vi "Autonomous Independent.vi"() -> ()   [LabVIEW 2016]
doc: "This VI is called when autonomous begins, and will automatically be terminated when autonomous ends. You can carry out timed or sensor driven robot movement independently without needing to return to the caller."
uses:
  <vilib>/Rock Robotics/Network Tables/NT Read Number.vi
  Global 2.vi
  Systems/Global 1.vi
panel:
  out "Numeric":i32=5
  out "Gyro":dbl=-2.5767482712972
  in  "Oscillate effort":dbl=0.25 format="%#_13g"
  out "Auto Mode":dbl
  in  "Auton_Modes":T1(array[cluster])=[{"Actions"=[{"Effort"=0.55, "Duration"=3.5, "Action"=enum."Vision Correction", "Encoder"=0.0, "Condition"=FALSE}, {"Effort"=0.0, "Duration"=0.0, "Action"=enum."Nothing", "Encoder"=0.0, "Condition"=FALSE}]}, {"Actions"=[{"Effort"=0.53, "Duration"=1.0, "Action"=enum."Shoot", "Encoder"=6.462, "Condition"=TRUE}, {"Effort"=0.0, "Duration"=3.0, "Action"=enum."Index", "Encoder"=0.0, "Condition"=FALSE}, {"Effort"=0.3, "Duration"=2.0, "Action"=enum."Turn", "Encoder"=38.0, "Condition"=FALSE}, {"Effort"=0.3, "Duration"=5.0, "Action"=enum."Drive", "Encoder"=0.0, "Condition"=TRUE}, {"Effort"=0.25, "Duration"=0.0, "Action"=enum."Nothing", "Encoder"=57.0, "Condition"=FALSE}, {"Effort"=-0.25, "Duration"=0.0, "Action"=enum."Nothing", "Encoder"=0.0, "Condition"=FALSE}, {"Effort"=1.0, "Duration"=0.0, "Action"=enum."Nothing", "Encoder"=0.0, "Condition"=FALSE}, {"Effort"=0.25, "Duration"=0.0, "Action"=enum."Nothing", "Encoder"=0.0, "Condition"=FALSE}]}, {"Actions"=[{"Effort"=0.0, "Duration"=0.1, "Action"=enum."Drive Encoder Reset", "Encoder"=0.0, "Condition"=FALSE}, {"Effort"=0.0, "Duration"=0.1, "Action"=enum."Gyro Reset", "Encoder"=0.0, "Condition"=FALSE}, {"Effort"=0.3, "Duration"=4.0, "Action"=enum."Drive", "Encoder"=60.0, "Condition"=FALSE}, {"Effort"=1.0, "Duration"=1.0, "Action"=enum."Gear0", "Encoder"=0.0, "Condition"=FALSE}, {"Effort"=1.0, "Duration"=0.0, "Action"=enum."Nothing", "Encoder"=0.0, "Condition"=FALSE}, {"Effort"=1.0, "Duration"=0.0, "Action"=enum."Nothing", "Encoder"=0.0, "Condition"=FALSE}, {"Effort"=0.0, "Duration"=0.0, "Action"=enum."Drive Encoder Reset", "Encoder"=0.0, "Condition"=FALSE}, {"Effort"=0.0, "Duration"=0.0, "Action"=enum."Nothing", "Encoder"=0.0, "Condition"=FALSE}, {"Effort"=0.0, "Duration"=0.0, "Action"=enum."Nothing", "Encoder"=0.0, "Condition"=FALSE}, {"Effort"=-0.2, "Duration"=10000.0, "Action"=enum."Drive", "Encoder"=24.0, "Condition"=FALSE}, {"Effort"=0.0, "Duration"=0.0, "Action"=enum."Drive Encoder Reset", "Encoder"=0.0, "Condition"=FALSE}, {"Effort"=-0.25, "Duration"=0.0, "Action"=enum."Nothing", "Encoder"=12.0, "Condition"=FALSE}]}, {"Actions"=[{"Effort"=0.0, "Duration"=0.1, "Action"=enum."Drive Encoder Reset", "Encoder"=6.462, "Condition"=FALSE}, {"Effort"=0.0, "Duration"=0.1, "Action"=enum."Gyro Reset", "Encoder"=0.0, "Condition"=FALSE}, {"Effort"=-0.25, "Duration"=1.0, "Action"=enum."Drive", "Encoder"=6.462, "Condition"=FALSE}, {"Effort"=0.0, "Duration"=0.1, "Action"=enum."Gyro Reset", "Encoder"=0.0, "Condition"=FALSE}, {"Effort"=-0.25, "Duration"=0.0, "Action"=enum."Turn", "Encoder"=0.0, "Condition"=FALSE}, {"Effort"=-0.25, "Duration"=0.0, "Action"=enum."Drive", "Encoder"=7.5, "Condition"=FALSE}, {"Effort"=-1.0, "Duration"=0.0, "Action"=enum."Gear0", "Encoder"=0.0, "Condition"=FALSE}, {"Effort"=0.25, "Duration"=0.0, "Action"=enum."Drive", "Encoder"=3.0, "Condition"=FALSE}]}, {"Actions"=[{"Effort"=0.0, "Duration"=0.1, "Action"=enum."Drive Encoder Reset", "Encoder"=6.462, "Condition"=FALSE}, {"Effort"=0.0, "Duration"=0.1, "Action"=enum."Gyro Reset", "Encoder"=0.0, "Condition"=FALSE}, {"Effort"=-0.25, "Duration"=1.0, "Action"=enum."Drive", "Encoder"=6.462, "Condition"=FALSE}, {"Effort"=0.0, "Duration"=0.1, "Action"=enum."Gyro Reset", "Encoder"=0.0, "Condition"=FALSE}, {"Effort"=-0.25, "Duration"=0.0, "Action"=enum."Turn", "Encoder"=0.0, "Condition"=FALSE}, {"Effort"=-0.25, "Duration"=0.0, "Action"=enum."Drive", "Encoder"=7.5, "Condition"=FALSE}, {"Effort"=-1.0, "Duration"=0.0, "Action"=enum."Gear0", "Encoder"=0.0, "Condition"=FALSE}, {"Effort"=0.25, "Duration"=0.0, "Action"=enum."Drive", "Encoder"=3.0, "Condition"=FALSE}]}, {"Actions"=[{"Effort"=0.0, "Duration"=0.1, "Action"=enum."Drive Encoder Reset", "Encoder"=0.0, "Condition"=FALSE}, {"Effort"=0.0, "Duration"=0.1, "Action"=enum."Gyro Reset", "Encoder"=0.0, "Condition"=FALSE}, {"Effort"=0.25, "Duration"=1.0, "Action"=enum."Drive", "Encoder"=6.462, "Condition"=FALSE}, {"Effort"=1.0, "Duration"=0.1, "Action"=enum."Gyro Reset", "Encoder"=0.0, "Condition"=FALSE}, {"Effort"=0.25, "Duration"=0.0, "Action"=enum."Turn", "Encoder"=0.0, "Condition"=FALSE}, {"Effort"=0.25, "Duration"=0.0, "Action"=enum."Drive", "Encoder"=7.5, "Condition"=FALSE}, {"Effort"=1.0, "Duration"=0.0, "Action"=enum."Gear0", "Encoder"=0.0, "Condition"=FALSE}, {"Effort"=-0.25, "Duration"=0.0, "Action"=enum."Drive", "Encoder"=3.0, "Condition"=FALSE}]}, {"Actions"=[{"Effort"=0.0, "Duration"=0.1, "Action"=enum."Nothing", "Encoder"=0.0, "Condition"=FALSE}, {"Effort"=0.0, "Duration"=0.1, "Action"=enum."Gyro Reset", "Encoder"=0.0, "Condition"=FALSE}, {"Effort"=0.25, "Duration"=5.0, "Action"=enum."Drive", "Encoder"=60000.0, "Condition"=TRUE}, {"Effort"=0.75, "Duration"=1.0, "Action"=enum."Nothing", "Encoder"=0.0, "Condition"=FALSE}, {"Effort"=0.0, "Duration"=1.0, "Action"=enum."Nothing", "Encoder"=0.0, "Condition"=FALSE}, {"Effort"=0.0, "Duration"=0.0, "Action"=enum."Nothing", "Encoder"=0.0, "Condition"=FALSE}]}, {"Actions"=[{"Effort"=0.0, "Duration"=0.1, "Action"=enum."Drive Encoder Reset", "Encoder"=0.0, "Condition"=FALSE}, {"Effort"=0.0, "Duration"=0.1, "Action"=enum."Gyro Reset", "Encoder"=0.0, "Condition"=FALSE}, {"Effort"=0.3, "Duration"=0.0, "Action"=enum."Drive", "Encoder"=24.0, "Condition"=FALSE}, {"Effort"=0.3, "Duration"=3.0, "Action"=enum."Nothing", "Encoder"=0.0, "Condition"=FALSE}, {"Effort"=0.3, "Duration"=2.0, "Action"=enum."Vision Correction", "Encoder"=30.0, "Condition"=FALSE}, {"Effort"=0.2, "Duration"=1.0, "Action"=enum."Drive", "Encoder"=18.5, "Condition"=TRUE}, {"Effort"=1.0, "Duration"=0.0, "Action"=enum."Gear0", "Encoder"=0.0, "Condition"=FALSE}, {"Effort"=-0.2, "Duration"=1.3, "Action"=enum."Drive", "Encoder"=30.0, "Condition"=TRUE}, {"Effort"=0.0, "Duration"=3.0, "Action"=enum."Nothing", "Encoder"=0.0, "Condition"=FALSE}, {"Effort"=0.03, "Duration"=0.0, "Action"=enum."Turn", "Encoder"=0.0, "Condition"=FALSE}, {"Effort"=0.0, "Duration"=0.0, "Action"=enum."Drive", "Encoder"=0.0, "Condition"=FALSE}]}, {"Actions"=[{"Effort"=0.0, "Duration"=0.0, "Action"=enum."Nothing", "Encoder"=0.0, "Condition"=FALSE}]}, {"Actions"=[{"Effort"=0.0, "Duration"=2.5, "Action"=enum."Shoot", "Encoder"=0.0, "Condition"=FALSE}, {"Effort"=0.0, "Duration"=5.0, "Action"=enum."Index", "Encoder"=0.0, "Condition"=FALSE}, {"Effort"=0.25, "Duration"=3.5, "Action"=enum."Nothing", "Encoder"=88.0, "Condition"=FALSE}, {"Effort"=1.0, "Duration"=1.0, "Action"=enum."Nothing", "Encoder"=0.0, "Condition"=FALSE}, {"Effort"=1.0, "Duration"=1.0, "Action"=enum."Nothing", "Encoder"=0.0, "Condition"=FALSE}, {"Effort"=1.0, "Duration"=0.5, "Action"=enum."Nothing", "Encoder"=0.0, "Condition"=FALSE}, {"Effort"=0.0, "Duration"=0.0, "Action"=enum."Nothing", "Encoder"=0.0, "Condition"=FALSE}, {"Effort"=-0.25, "Duration"=0.0, "Action"=enum."Nothing", "Encoder"=3.0, "Condition"=FALSE}, {"Effort"=0.0, "Duration"=0.0, "Action"=enum."Nothing", "Encoder"=0.0, "Condition"=FALSE}, {"Effort"=0.25, "Duration"=0.0, "Action"=enum."Nothing", "Encoder"=24.0, "Condition"=FALSE}, {"Effort"=0.0, "Duration"=0.0, "Action"=enum."Nothing", "Encoder"=0.0, "Condition"=FALSE}, {"Effort"=-0.25, "Duration"=0.0, "Action"=enum."Nothing", "Encoder"=12.0, "Condition"=FALSE}]}, {"Actions"=[{"Effort"=0.0, "Duration"=0.1, "Action"=enum."Drive Encoder Reset", "Encoder"=0.0, "Condition"=FALSE}, {"Effort"=0.0, "Duration"=1.0, "Action"=enum."Gyro Reset", "Encoder"=0.0, "Condition"=FALSE}, {"Effort"=0.3, "Duration"=1.4, "Action"=enum."Drive", "Encoder"=88.0, "Condition"=FALSE}, {"Effort"=0.3, "Duration"=3.0, "Action"=enum."Turn", "Encoder"=2.0, "Condition"=FALSE}, {"Effort"=1.0, "Duration"=1.0, "Action"=enum."Nothing", "Encoder"=0.0, "Condition"=FALSE}, {"Effort"=1.0, "Duration"=1.0, "Action"=enum."Nothing", "Encoder"=0.0, "Condition"=FALSE}, {"Effort"=0.0, "Duration"=0.0, "Action"=enum."Nothing", "Encoder"=0.0, "Condition"=FALSE}, {"Effort"=-0.25, "Duration"=0.0, "Action"=enum."Nothing", "Encoder"=3.0, "Condition"=FALSE}, {"Effort"=0.0, "Duration"=0.0, "Action"=enum."Nothing", "Encoder"=0.0, "Condition"=FALSE}, {"Effort"=0.25, "Duration"=0.0, "Action"=enum."Nothing", "Encoder"=24.0, "Condition"=FALSE}, {"Effort"=0.0, "Duration"=0.0, "Action"=enum."Nothing", "Encoder"=0.0, "Condition"=FALSE}, {"Effort"=-0.25, "Duration"=0.0, "Action"=enum."Nothing", "Encoder"=12.0, "Condition"=FALSE}]}, {"Actions"=[{"Effort"=0.0, "Duration"=1.0, "Action"=enum."Drive Encoder Reset", "Encoder"=0.0, "Condition"=FALSE}, {"Effort"=0.0, "Duration"=1.0, "Action"=enum."Shoot", "Encoder"=0.0, "Condition"=FALSE}, {"Effort"=0.25, "Duration"=5.0, "Action"=enum."Index", "Encoder"=88.0, "Condition"=FALSE}, {"Effort"=1.0, "Duration"=1.0, "Action"=enum."Nothing", "Encoder"=0.0, "Condition"=FALSE}, {"Effort"=1.0, "Duration"=1.0, "Action"=enum."Nothing", "Encoder"=0.0, "Condition"=FALSE}, {"Effort"=1.0, "Duration"=0.5, "Action"=enum."Nothing", "Encoder"=0.0, "Condition"=FALSE}, {"Effort"=0.0, "Duration"=0.0, "Action"=enum."Nothing", "Encoder"=0.0, "Condition"=FALSE}, {"Effort"=-0.25, "Duration"=0.0, "Action"=enum."Nothing", "Encoder"=3.0, "Condition"=FALSE}, {"Effort"=0.0, "Duration"=0.0, "Action"=enum."Nothing", "Encoder"=0.0, "Condition"=FALSE}, {"Effort"=0.25, "Duration"=0.0, "Action"=enum."Nothing", "Encoder"=24.0, "Condition"=FALSE}, {"Effort"=0.0, "Duration"=0.0, "Action"=enum."Nothing", "Encoder"=0.0, "Condition"=FALSE}, {"Effort"=-0.25, "Duration"=0.0, "Action"=enum."Nothing", "Encoder"=12.0, "Condition"=FALSE}]}, {"Actions"=[{"Effort"=0.0, "Duration"=0.1, "Action"=enum."Drive Encoder Reset", "Encoder"=0.0, "Condition"=FALSE}, {"Effort"=0.0, "Duration"=1.0, "Action"=enum."Gyro Reset", "Encoder"=0.0, "Condition"=FALSE}, {"Effort"=0.3, "Duration"=1.4, "Action"=enum."Drive", "Encoder"=88.0, "Condition"=FALSE}, {"Effort"=0.3, "Duration"=4.0, "Action"=enum."Turn", "Encoder"=0.0, "Condition"=FALSE}, {"Effort"=1.0, "Duration"=1.0, "Action"=enum."Nothing", "Encoder"=0.0, "Condition"=FALSE}, {"Effort"=1.0, "Duration"=0.5, "Action"=enum."Nothing", "Encoder"=0.0, "Condition"=FALSE}, {"Effort"=0.0, "Duration"=0.0, "Action"=enum."Nothing", "Encoder"=0.0, "Condition"=FALSE}, {"Effort"=0.3, "Duration"=0.5, "Action"=enum."Nothing", "Encoder"=24.0, "Condition"=TRUE}, {"Effort"=0.0, "Duration"=0.0, "Action"=enum."Nothing", "Encoder"=0.0, "Condition"=FALSE}, {"Effort"=-0.2, "Duration"=2.0, "Action"=enum."Nothing", "Encoder"=24.0, "Condition"=TRUE}, {"Effort"=0.0, "Duration"=0.0, "Action"=enum."Nothing", "Encoder"=0.0, "Condition"=FALSE}, {"Effort"=-0.25, "Duration"=0.0, "Action"=enum."Nothing", "Encoder"=12.0, "Condition"=FALSE}]}]
  # "Nothing"
  # "Boiler Right Right side gear"
  # "Middle Gear"
  # "Boiler Right Left Side Gear"
  # "Boiler Left RightSide Gear"
  # "Boiler Left Left Side Gear"
  # "Drive"
  # "Vision Correction"
  # "Hopper"
  # "10 ball"
  # "Farside"
  # "Boilerside-10 ball"
  # "Auto 5"
  # "Auto 6"
  # "Auto 6"
  # "Auto 7"
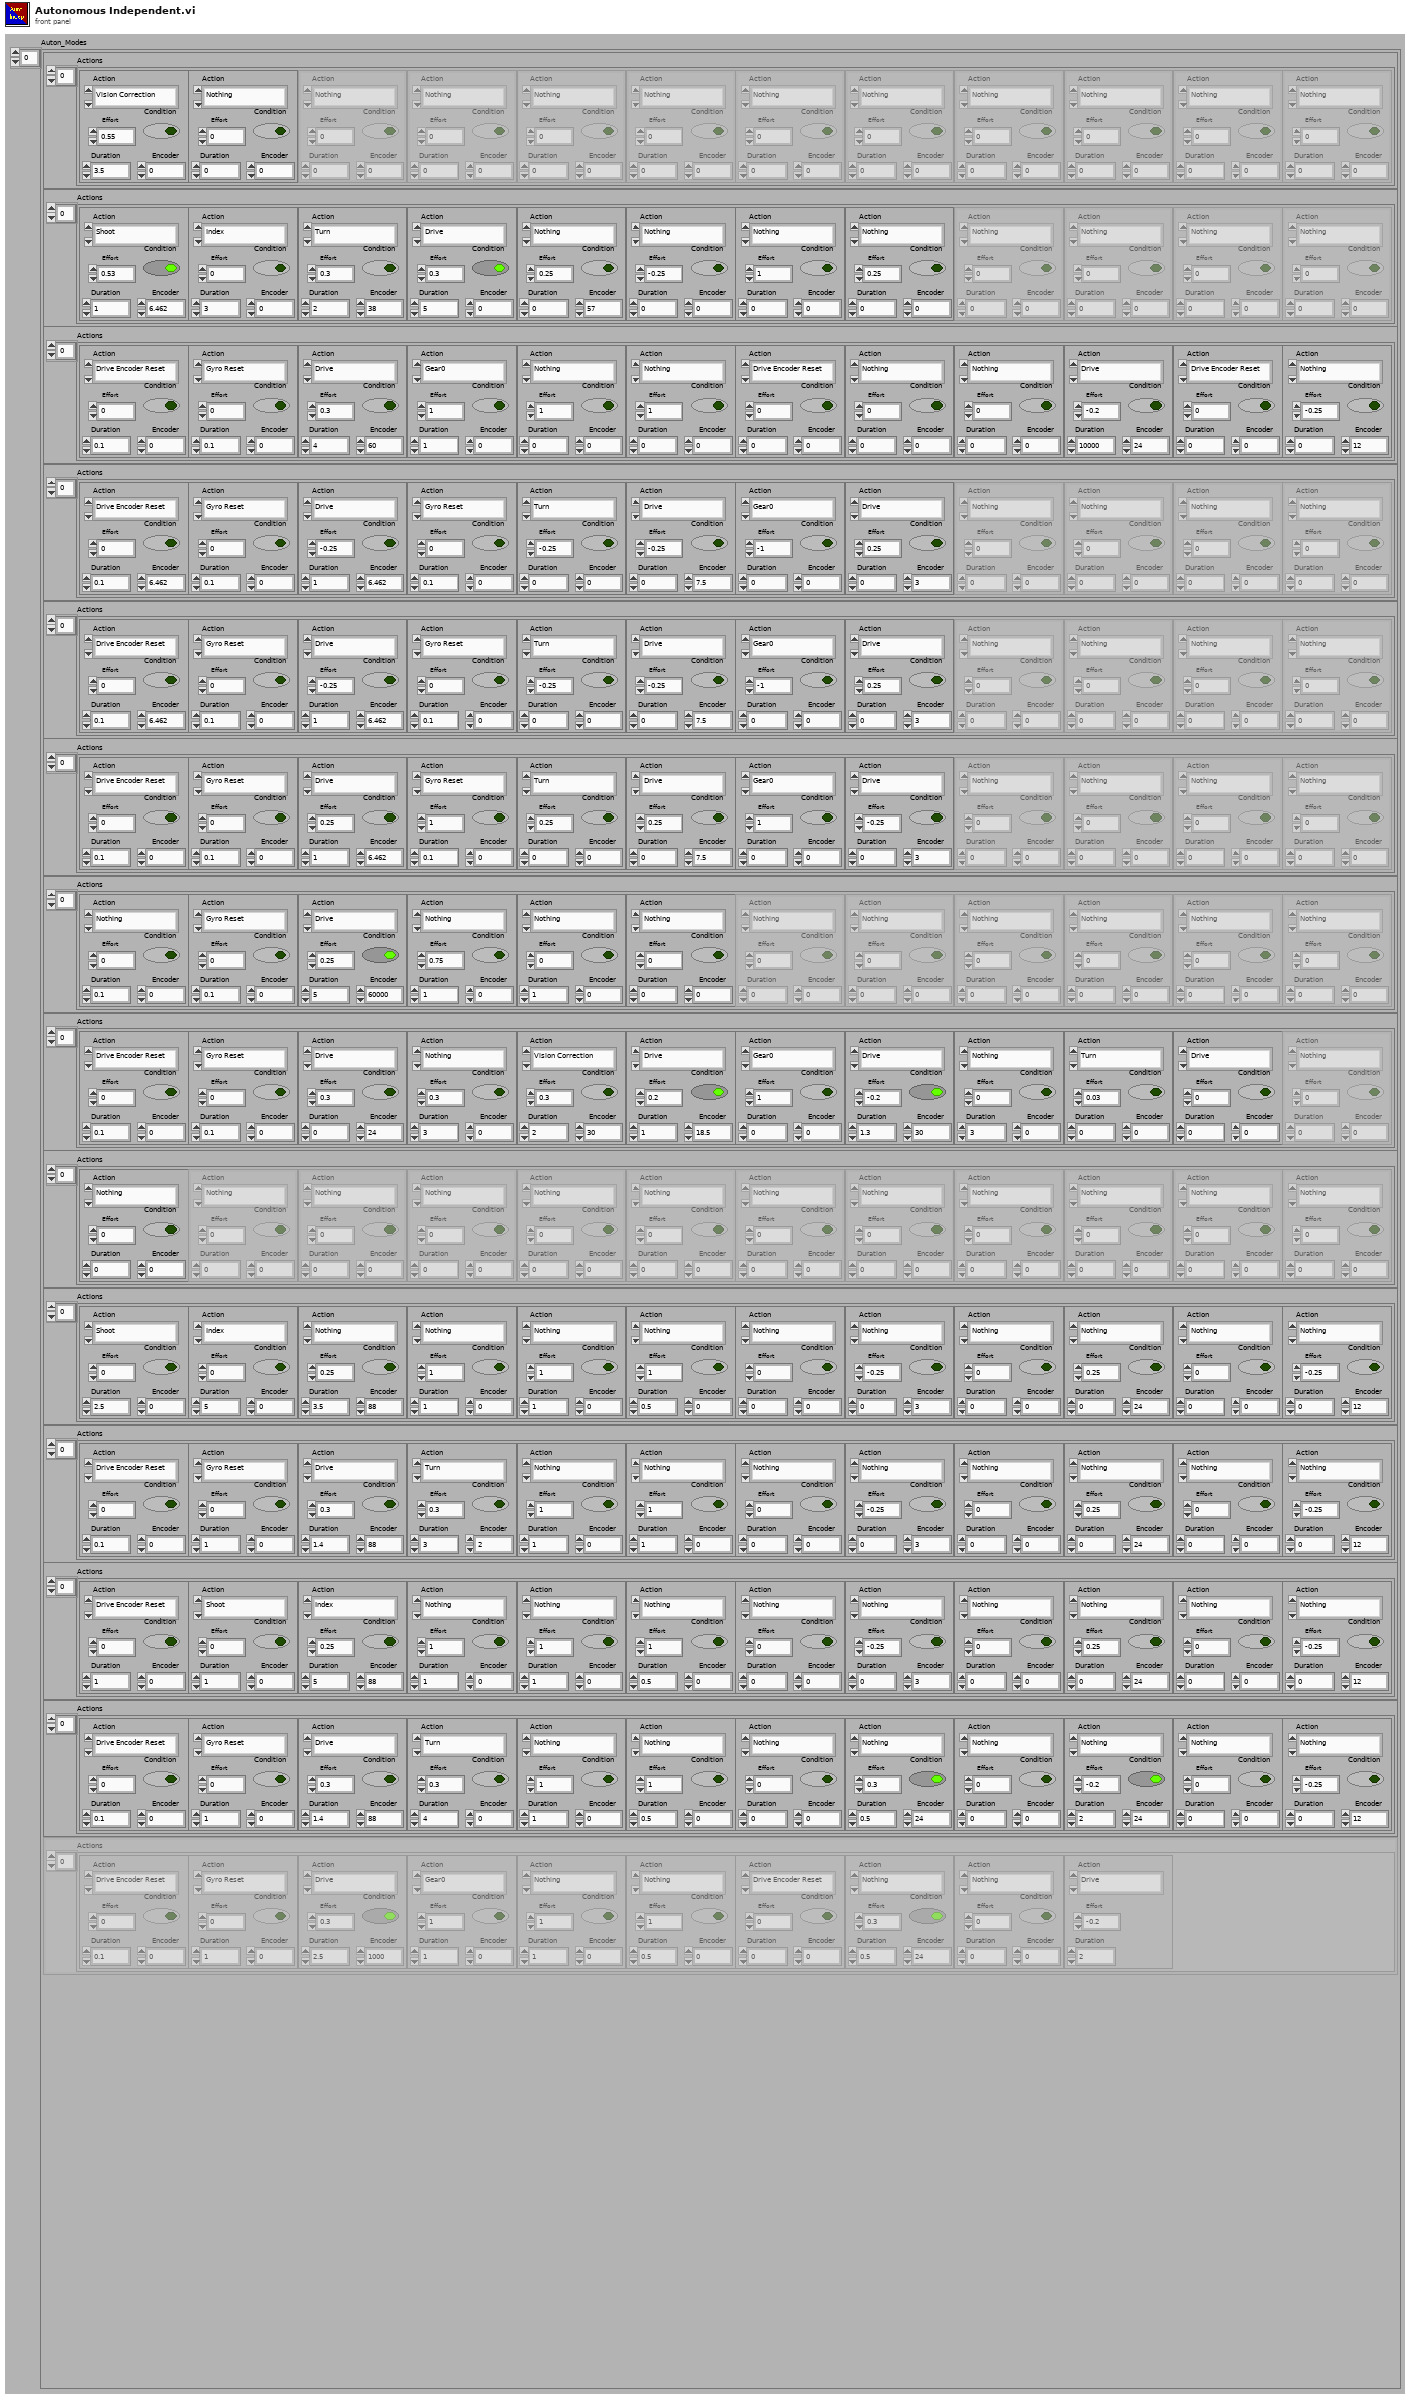
[diagram p1: front panel]
types:
  T1 = cluster{"Actions":cluster{"Effort":dbl, "Duration":dbl, "Action":enum16{"Nothing", "Drive", "Vision Correction", "Turn", "Gear0", "Gear1", "Climb", "Intake", "Index", "Shoot", "Test", "Drive Encoder Reset", "Gyro Reset"}, "Encoder":dbl, "Condition":bool}[]}[]
  T2 = cluster{"Actions":cluster{"Effort":dbl, "Duration":dbl, "Action":enum16{"Nothing", "Drive", "Vision Correction", "Turn", "Gear0", "Gear1", "Climb", "Intake", "Index", "Shoot", "Test", "Drive Encoder Reset", "Gyro Reset"}, "Encoder":dbl, "Condition":bool}[]}
  T3 = cluster{"Effort":dbl, "Duration":dbl, "Action":enum16{"Nothing", "Drive", "Vision Correction", "Turn", "Gear0", "Gear1", "Climb", "Intake", "Index", "Shoot", "Test", "Drive Encoder Reset", "Gyro Reset"}, "Encoder":dbl, "Condition":bool}[]
  T4 = enum16{"Nothing", "Drive", "Vision Correction", "Turn", "Gear0", "Gear1", "Climb", "Intake", "Index", "Shoot", "Test", "Drive Encoder Reset", "Gyro Reset"}
  T5 = typedef "WPI_MotorControlDeviceRef.ctl" = cluster{"DeviceStatus":errorcluster, "Type":T6, "PWM":cluster{"PWM Channel":T7, "DeadBand":T8}, "CAN":cluster{"Device Number":u8, "SetOutput VI Ref":variant, "GetOutput VI Ref":variant, "Enable VI Ref":variant, "Disable VI Ref":variant, "Data":variant}, "Invert":bool}
  T6 = typedef "WPI_MotorControlType.ctl" = enum16{"PWM", "CAN"}
  T7 = typedef "FPGA_DIOPWMChannel.ctl" = enum8{"PWM 0", "PWM 1", "PWM 2", "PWM 3", "PWM 4", "PWM 5", "PWM 6", "PWM 7", "PWM 8", "PWM 9", "PWM MXP 0", "PWM MXP 1", "PWM MXP 2", "PWM MXP 3", "PWM MXP 4", "PWM MXP 5", "PWM MXP 6", "PWM MXP 7", "PWM MXP 8", "PWM MXP 9", "Invalid"}
  T8 = typedef "WPI_PWMDeadband.ctl" = cluster{"Name":string, "maxPositivePwm":i32, "minPositivePwm":i32, "centerPwm":i32, "maxNegativePwm":i32, "minNegativePwm":i32, "angularRange":u16}
  T9 = typedef "WPI_CANTalonSRX_GlobalStatus.ctl" = cluster{"Applied Throttle":dbl, "Module Enabled":bool, "CAN Error":errorcluster, "Closed Loop Error":dbl, "Forward Limit Switch Closed":bool, "Reverse Limit Switch Closed":bool, "Sensor Position":dbl, "Sensor Velocity":dbl, "Current":dbl, "Sticky Fault - Over Temp":bool, "Sticky Fault - Under Voltage":bool, "Sticky Fault - Forward Limit":bool, "Sticky Fault - Reverse Limit":bool, "Sticky Fault - Forward Soft Limit":bool, "Sticky Fault - Reverse Soft Limit":bool, "Brake is Enabled":bool, "Encoder Position":dbl, "Encoder Velocity":dbl, "Encoder Index Count":dbl, "Encoder A Pin State":bool, "Encoder B Pin State":bool, "Encoder Index Pin State":bool, "Analog In":dbl, "Analog In Velocity":dbl, "Temperature (C)":dbl, "Battery Voltage":dbl, "Control 5 Is Supported":bool, "Current Profile Slot Select":dbl, "Pos Div 8":bool, "Vel Div 4":bool, "Pulse Width Position":i32, "Pulse Width Velocity":i32, "Pulse Width Rise To Rise (us)":i32, "Pulse Width Rise To Fall (us)":i32, "Mot Prof Active Is Under Run":bool, "Mot Prof Active Has Under Run":bool, "Mot Prof Active Is Last":bool, "Mot Prof Active Velocity Only":bool, "Mot Prof Active Is Valid":bool, "Mot Prof Buffer Is Full":bool, "Mot Prof Active Profile Slot Select":i32, "Mot Prof NextID":i32, "Mot Prof Count":i32, "Mot Prof Active Velocity":dbl, "Mot Prof Active Position":dbl, "Mot Prof Output Enable":i32}
  T10 = typedef "WPI_GyroDevRef.ctl" = cluster{"DevStatus":errorcluster, "Analog Channel":T11, "Offset":dbl, "Gain (VoltsPerDegree/Second)":dbl, "Gyro Type":enum16{"Analog", "XRS450"}, "Handle":i32, "SPI Bus":T12, "Device Found":bool, "Sample Rate":dbl, "Calibrate On Open":bool}
  T11 = typedef "FPGA_AIChannel.ctl" = enum8{"AI 0", "AI 1", "AI 2", "AI 3", "AI MXP 0", "AI MXP 1", "AI MXP 2", "AI MXP 3", "Invalid"}
  T12 = typedef "spi_bus.ctl" = enum16{"SPI On-Board, CS0", "SPI On-Board, CS1", "SPI On-Board, CS2", "SPI On-Board, CS3", "SPI MXP", "Invalid"}
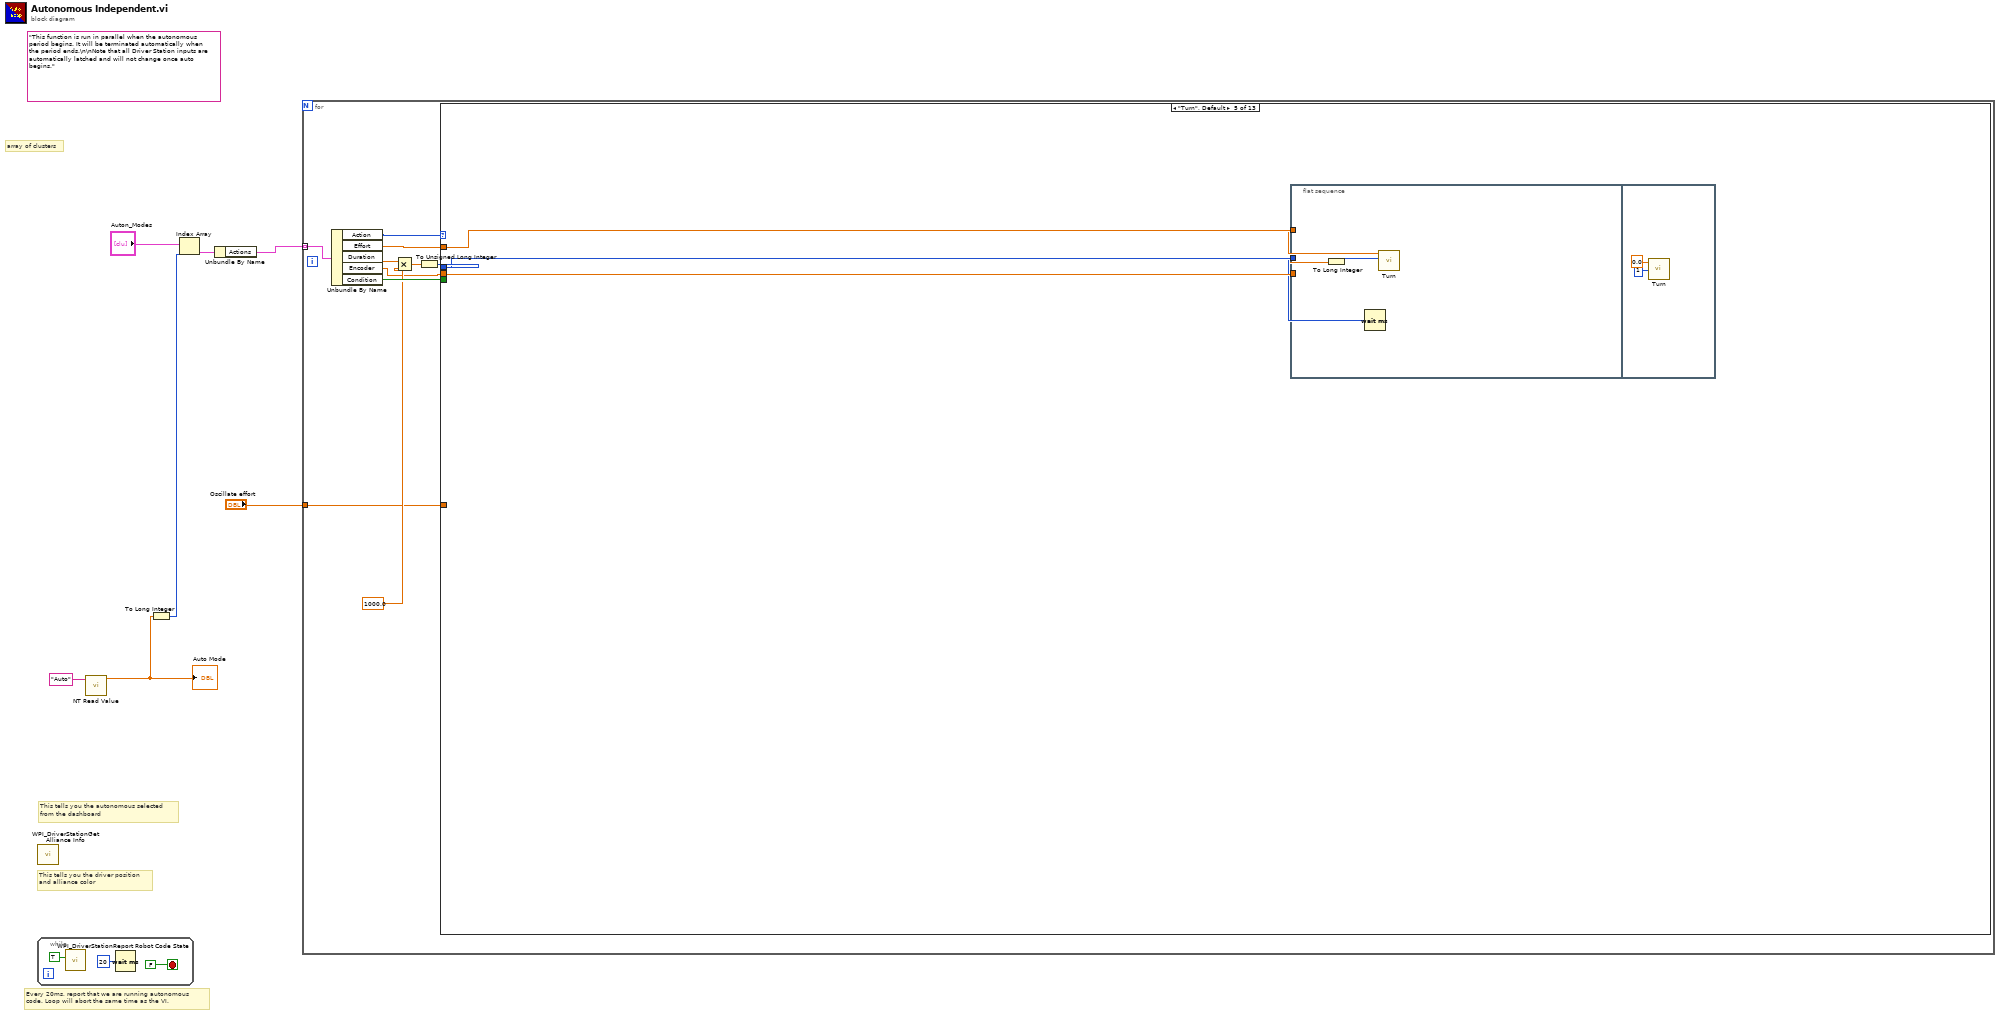
[diagram p0: block diagram]
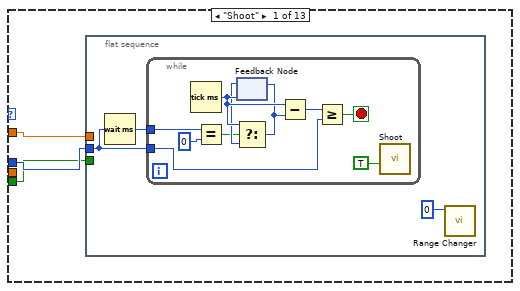
[diagram p2: hidden frame]
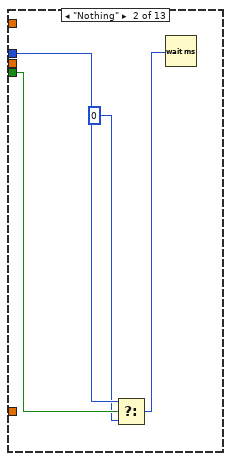
[diagram p3: hidden frame]
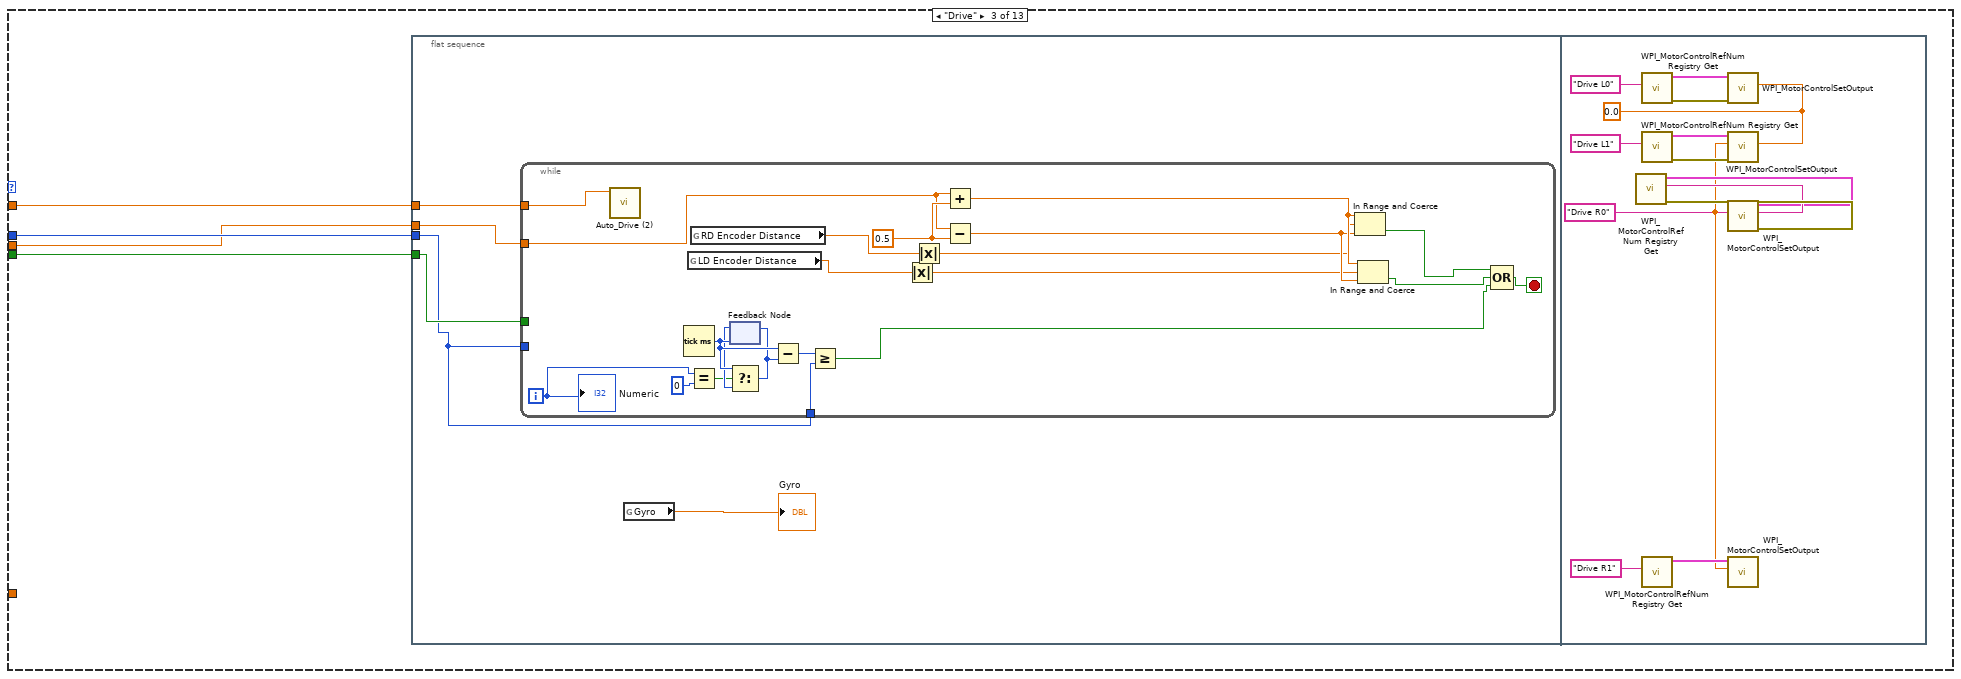
[diagram p4: hidden frame]
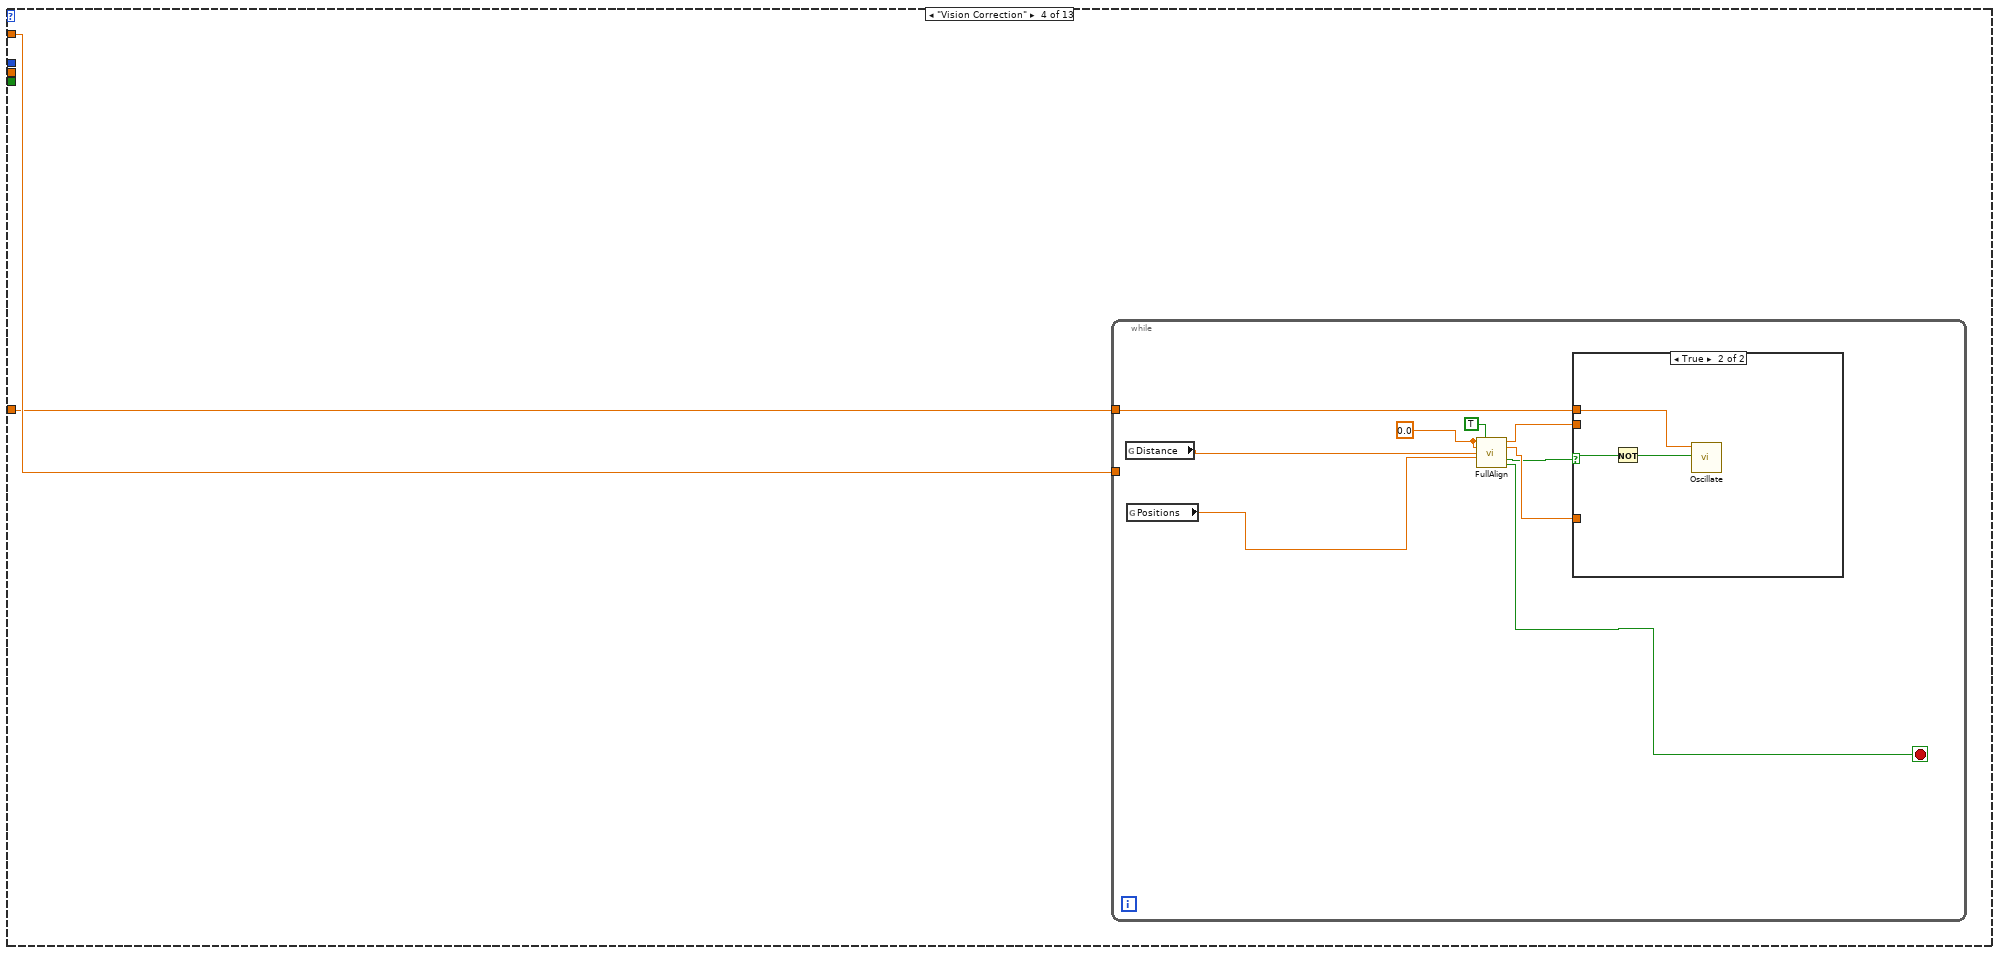
[diagram p5: hidden frame]
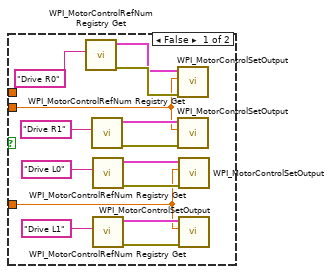
[diagram p6: hidden frame]
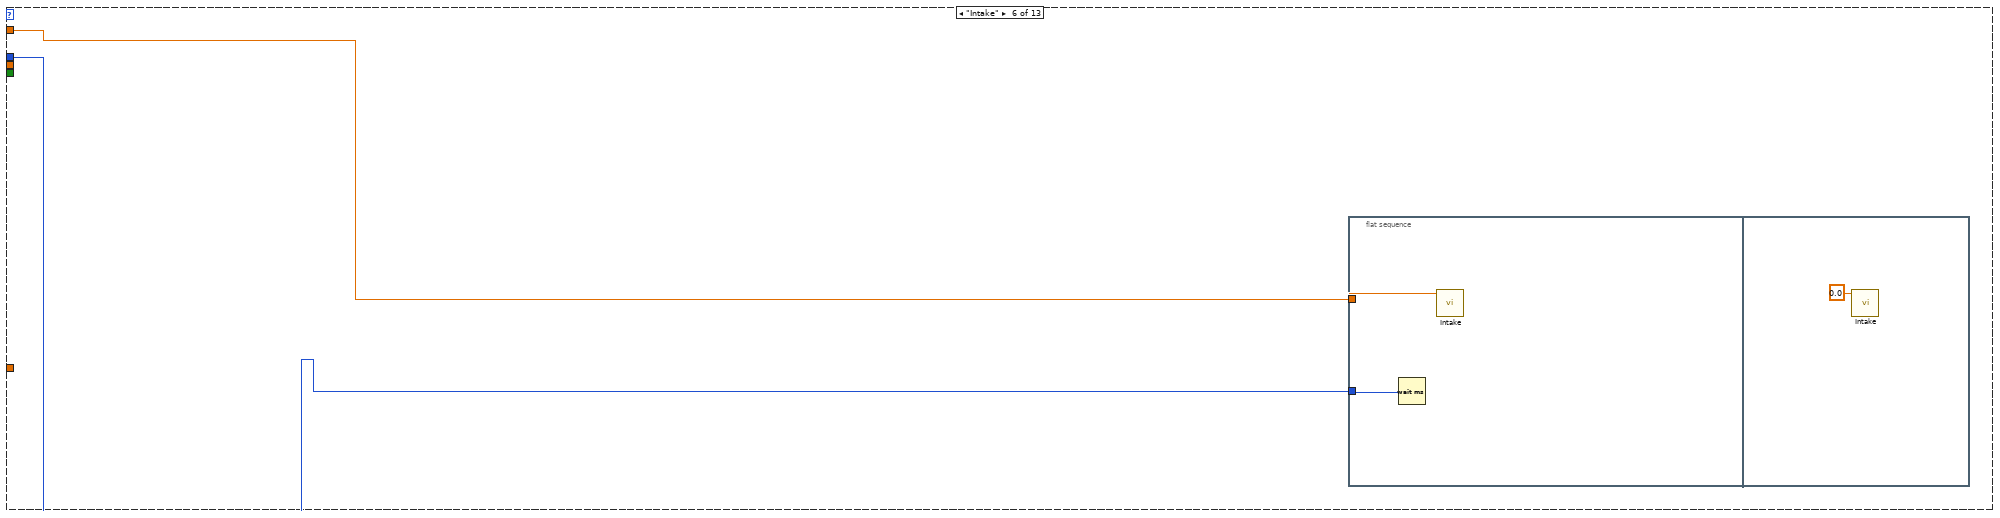
[diagram p7: hidden frame]
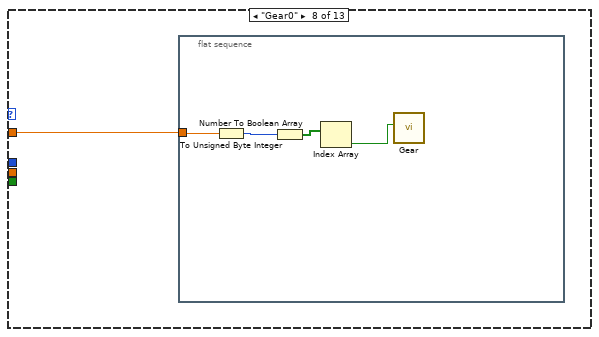
[diagram p9: hidden frame]
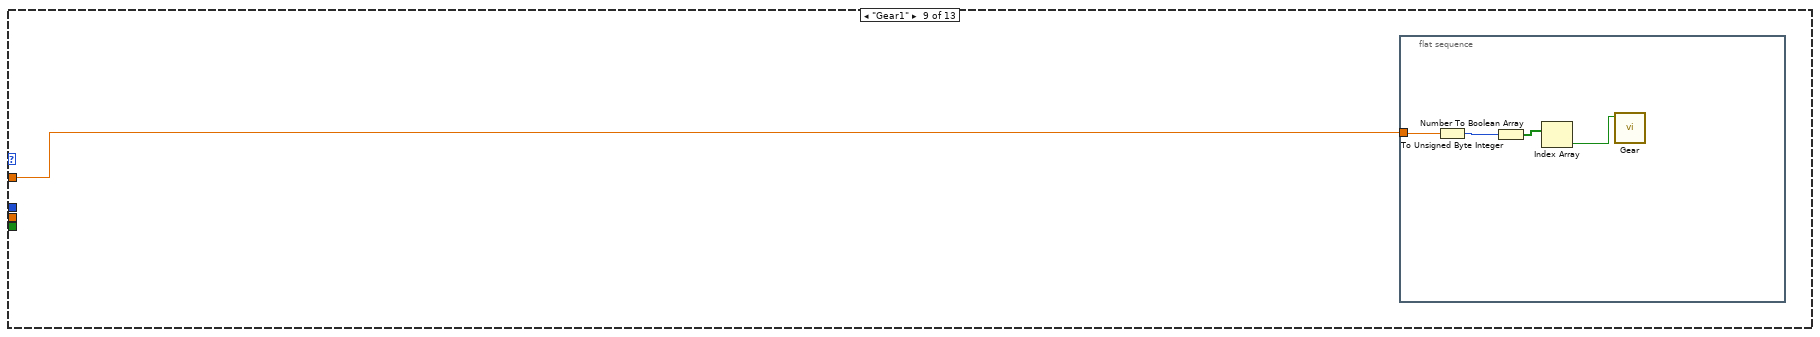
[diagram p10: hidden frame]
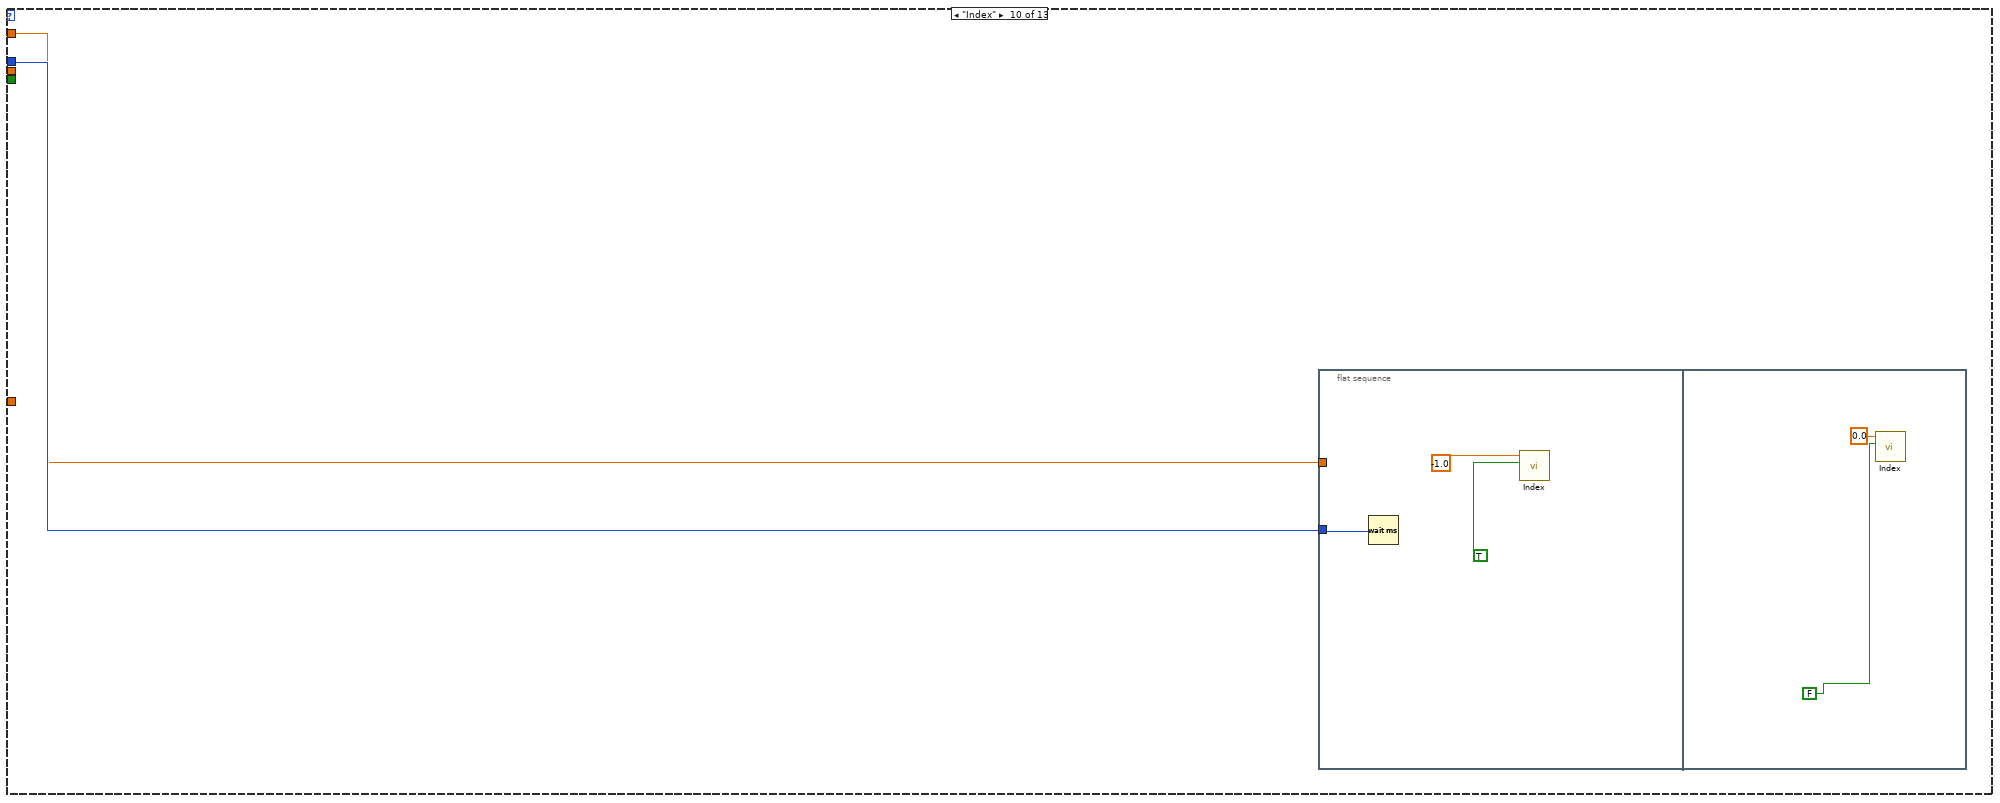
[diagram p11: hidden frame]
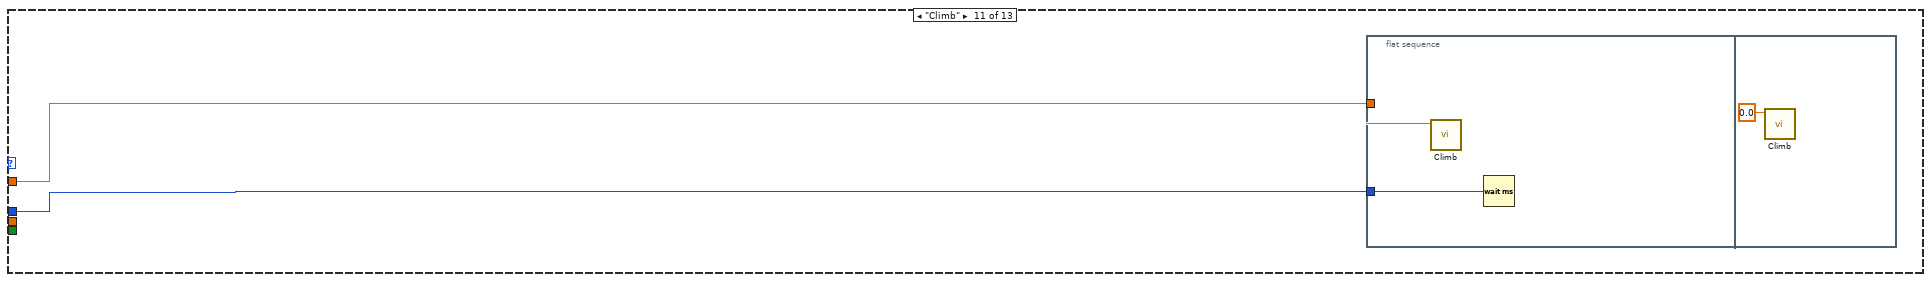
[diagram p12: hidden frame]
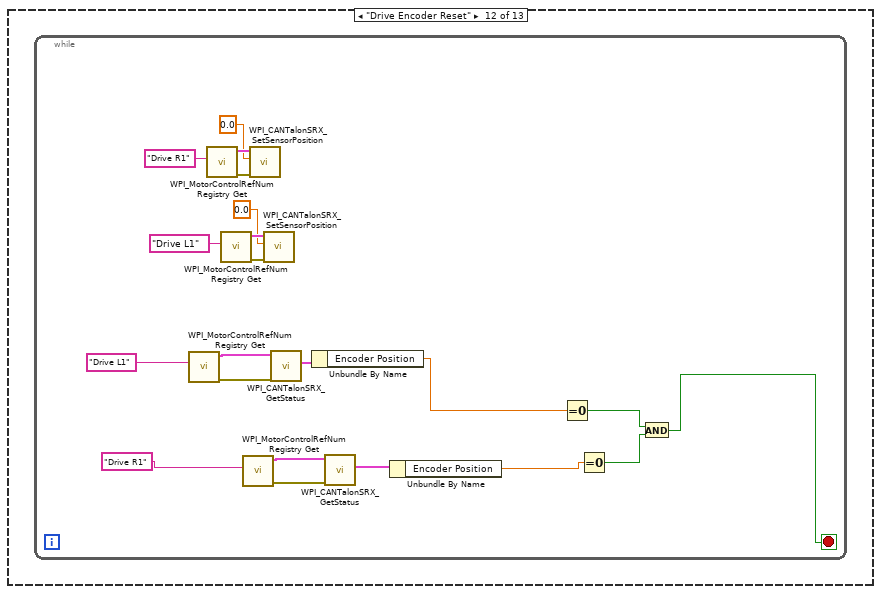
[diagram p13: hidden frame]
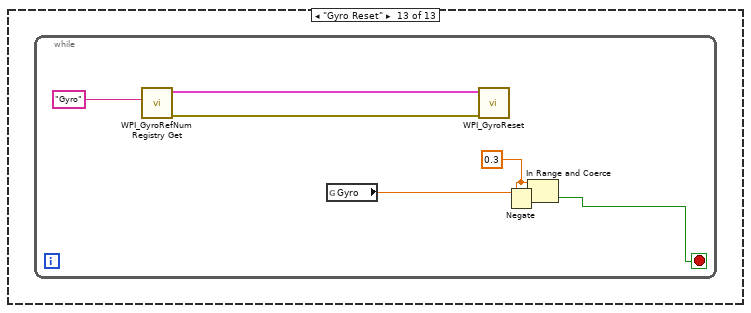
[diagram p14: hidden frame]
diagram:
  (unwired) "This function is run in parallel when the autonomous period begins. It will be terminated automatically when the period ends.\n\nNote that all Driver Station inputs are automatically latched and will not change once auto begins."
  # "This tells you the autonomous selected\nfrom the dashboard"
  # "array of clusters"
  # "Every 20ms, report that we are running autonomous\ncode. Loop will abort the same time as the VI."
  # "This tells you the driver position\nand alliance color"
  n1 = while {
    stop <- FALSE stop-if-true
    n2 = call <vilib>:"WPI_DriverStationReport Robot Code State.vi"("Autonomous"=TRUE) -> ()  [unwired: 10 in, 1 out]
    n3 = Wait (ms)(milliseconds to wait=u32 20) -> ()  [unwired: 1 out]
  }
  n4 = call <vilib>:"WPI_DriverStationGet Alliance Info.vi"() -> ()  [unwired: 12 out]
  n5 = call-poly <vilib>:"NT Read Value.vi"("Name"="Auto") -> ("Numeric"=w2:dbl)  [unwired: 9 in, 1 out]
  "Auto Mode" <- w2
  n6 = To Long Integer(number=w2) -> (32bit integer=w4:i32)
  n7 = Index Array(array="Auton_Modes", index=w4) -> (element=w6:T2)
  n8 = Unbundle By Name(w6) -> ("Actions"=w7:T3)
  n9 = for {
    tunnel: w7 -> [w20] mode=indexing
    tunnel: "Oscillate effort" -> [w12]
    n10 = Unbundle By Name(w20) -> ("Action"=w11:T4, "Effort"=w19:dbl, "Duration"=w18:dbl, "Encoder"=w13:dbl, "Condition"=w15:bool)
    n11 = Multiply(x=w18, y=1000.0) -> (x*y=w17:dbl)
    n12 = To Unsigned Long Integer(number=w17) -> (unsigned 32bit integer=w16:u32)
    n13 = case shown="\"Turn\", Default" w11 {
      tunnel: w19 -> [w23 _ w44 w84 w113 w121 _ w125 w130 w135 w143 _ _]
      tunnel: w16 -> [w22 w39 w43 _ w112 w120 _ _ _ w136 w142 _ _]
      tunnel: w15 -> [w21 w40 w42 _ _ _ _ _ _ _ _ _ _]
      tunnel: w13 -> [_ _ w41 _ w111 _ _ _ _ _ _ _ _]
      tunnel: w12 -> [_ _ _ w83 _ _ _ _ _ _ _ _ _]
      frame "Shoot" {
        n14 = flat-sequence {
          tunnel: w23 -> [_]
          tunnel: w22 -> [w24]
          tunnel: w21 -> [_]
          frame #0 {
            n15 = Wait (ms)(milliseconds to wait=w24) -> (millisecond timer value=w25:u32)
            n16 = while {
              tunnel: w25 -> [w28]
              tunnel: w24 -> [w27]
              stop <- w29 stop-if-true
              n17 = Tick Count (ms)() -> (millisecond timer value=w35:u32)
              n18 = Equal?(x=w28, y=0) -> (x = y?=w33:bool)
              n19 = feedback #1(w35) -> (w34:u32)
              n20 = Select(t=w35, s=w33, f=w34) -> (s? t:f=w31:u32)
              n21 = feedback-in #1(w31) -> ()
              n22 = Subtract(x=w35, y=w31) -> (x-y=w30:u32)
              n23 = Greater Or Equal?(x=w30, y=w27) -> (x >= y?=w29:bool)
              n24 = call "Shoot.vi"("Shoot"=TRUE) -> ()  [unwired: 10 in]
            }
            n25 = call "Range Changer.vi"("POV"=i16 0) -> ()  [unwired: 10 in, 1 out]
          }
        }
      }
      frame "Nothing" {
        n26 = Select(t=w39, s=w40, f=u32 0) -> (s? t:f=w37:u32)
        n27 = Wait (ms)(milliseconds to wait=w37) -> ()  [unwired: 1 out]
      }
      frame "Drive" {
        n28 = flat-sequence {
          tunnel: w44 -> [w49]
          tunnel: w43 -> [w45]
          tunnel: w42 -> [w47]
          tunnel: w41 -> [w48]
          frame #0 {
            n29 = while {
              tunnel: w49 -> [w70]
              tunnel: w48 -> [w60]
              tunnel: w47 -> [_]
              tunnel: w45 -> [_]
              tunnel: w45 -> [w63]
              i -> [w62]
              stop <- w52 stop-if-true
              w61 = 0.5 ("Range")
              n30 = call "Auto_Drive (2).vi"("Drive Effort"=w70) -> ()  [unwired: 11 in]
              n31 = Tick Count (ms)() -> (millisecond timer value=w69:u32)
              n32 = global read "Global 2.vi" "LD Encoder Distance"() -> (w56:dbl)
              n33 = Equal?(x=w62, y=0) -> (x = y?=w67:bool)
              n34 = global read "Global 2.vi" "RD Encoder Distance"() -> (w57:dbl)
              n35 = feedback #2(w69) -> (w68:u32)
              n36 = Select(t=w69, s=w67, f=w68) -> (s? t:f=w65:u32)
              n37 = feedback-in #2(w65) -> ()
              n38 = Subtract(x=w69, y=w65) -> (x-y=w64:u32)
              n39 = Greater Or Equal?(x=w64, y=w63) -> (x >= y?=w55:bool)
              n40 = Absolute Value(x=w56) -> (abs(x)=w50:dbl)
              n41 = Absolute Value(x=w57) -> (abs(x)=w51:dbl)
              n42 = Add(x=w60, y=w61) -> (x+y=w59:dbl)
              n43 = Subtract(x=w60, y=w61) -> (x-y=w58:dbl)
              n44 = In Range and Coerce(upper limit=w59, x=w51, lower limit=w58) -> (In Range?=w53:bool)  [unwired: 1 out]
              n45 = In Range and Coerce(upper limit=w59, x=w50, lower limit=w58) -> (In Range?=w54:bool)  [unwired: 1 out]
              n46 = Compound Arithmetic op=OR(w53, w54, w55) -> (w52:bool)
              "Numeric" <- w62
            }
            n47 = global read "Global 2.vi" "Gyro"() -> (→"Gyro":dbl)
          }
          frame #1 {
            w71 = 0.0 ("Drive L")
            n48 = call <vilib>:"WPI_MotorControlRefNum Registry Get.vi"("refnum name"="Drive R0") -> ("error out"=w76:errorcluster, "MotorControlDevRef"=w72:T5)  [unwired: 9 in]
            n49 = call <vilib>:"WPI_MotorControlRefNum Registry Get.vi"("refnum name"="Drive L0") -> ("error out"=w77:errorcluster, "MotorControlDevRef"=w78:T5)  [unwired: 9 in]
            n50 = call <vilib>:"WPI_MotorControlRefNum Registry Get.vi"("refnum name"="Drive L1") -> ("error out"=w81:errorcluster, "MotorControlDevRef"=w80:T5)  [unwired: 9 in]
            n51 = call <vilib>:"WPI_MotorControlRefNum Registry Get.vi"("refnum name"="Drive R1") -> ("MotorControlDevRef"=w74:T5)  [unwired: 9 in, 1 out]
            n52 = call <vilib>:"WPI_MotorControlSetOutput.vi"("error in (no error)"=w77, "Output"=w71, "MotorControlDevRef"=w78) -> ()  [unwired: 6 in, 3 out]
            n53 = call <vilib>:"WPI_MotorControlSetOutput.vi"("error in (no error)"=w81, "Output"=w71, "MotorControlDevRef"=w80) -> ()  [unwired: 6 in, 3 out]
            n54 = call <vilib>:"WPI_MotorControlSetOutput.vi"("error in (no error)"=w76, "Output"=w71, "MotorControlDevRef"=w72) -> ()  [unwired: 6 in, 3 out]
            n55 = call <vilib>:"WPI_MotorControlSetOutput.vi"("Output"=w71, "MotorControlDevRef"=w74) -> ()  [unwired: 7 in, 3 out]
          }
        }
      }
      frame "Vision Correction" {
        n56 = while {
          tunnel: w84 -> [_]
          tunnel: w83 -> [w87]
          stop <- w88 stop-if-true
          w91 = 0.0
          n57 = global read "Global 1.vi" "Distance"() -> (w90:dbl)
          n58 = global read "Global 1.vi" "Positions"() -> (w89:dbl)
          n59 = call "FullAlign.vi"("Joystick 0"=w91, "Button"=TRUE, "Joystick 1"=w91, "Distance"=w90, "Angle"=w89) -> ("Right Motor"=w93:dbl, "Left Motor"=w92:dbl, "Not In Sight?"=w85:bool, "In Range?"=w88:bool)  [unwired: 7 in]
          n60 = case shown="True" w85 {
            selector: w85 -> [_ w110]
            tunnel: w93 -> [w95 _]
            tunnel: w92 -> [w94 _]
            tunnel: w87 -> [_ w108]
            frame False {
              n61 = call <vilib>:"WPI_MotorControlRefNum Registry Get.vi"("refnum name"="Drive R0") -> ("error out"=w101:errorcluster, "MotorControlDevRef"=w97:T5)  [unwired: 9 in]
              n62 = call <vilib>:"WPI_MotorControlRefNum Registry Get.vi"("refnum name"="Drive R1") -> ("error out"=w96:errorcluster, "MotorControlDevRef"=w99:T5)  [unwired: 9 in]
              n63 = call <vilib>:"WPI_MotorControlRefNum Registry Get.vi"("refnum name"="Drive L0") -> ("error out"=w102:errorcluster, "MotorControlDevRef"=w103:T5)  [unwired: 9 in]
              n64 = call <vilib>:"WPI_MotorControlRefNum Registry Get.vi"("refnum name"="Drive L1") -> ("error out"=w106:errorcluster, "MotorControlDevRef"=w105:T5)  [unwired: 9 in]
              n65 = call <vilib>:"WPI_MotorControlSetOutput.vi"("error in (no error)"=w101, "Output"=w95, "MotorControlDevRef"=w97) -> ()  [unwired: 6 in, 3 out]
              n66 = call <vilib>:"WPI_MotorControlSetOutput.vi"("error in (no error)"=w96, "Output"=w95, "MotorControlDevRef"=w99) -> ()  [unwired: 6 in, 3 out]
              n67 = call <vilib>:"WPI_MotorControlSetOutput.vi"("error in (no error)"=w102, "Output"=w94, "MotorControlDevRef"=w103) -> ()  [unwired: 6 in, 3 out]
              n68 = call <vilib>:"WPI_MotorControlSetOutput.vi"("error in (no error)"=w106, "Output"=w94, "MotorControlDevRef"=w105) -> ()  [unwired: 6 in, 3 out]
            }
            frame True {
              n69 = Not(x=w110) -> (.not. x?=w109:bool)
              n70 = call "Oscillate.vi"("Target In Sight?"=w109, "Effort"=w108) -> ()  [unwired: 10 in]
            }
          }
        }
      }
      frame "Turn", Default {
        n71 = flat-sequence {
          tunnel: w113 -> [w117]
          tunnel: w112 -> [w116]
          tunnel: w111 -> [w114]
          frame #0 {
            n72 = To Long Integer(number=w114) -> (32bit integer=w115:i32)
            n73 = Wait (ms)(milliseconds to wait=w116) -> ()  [unwired: 1 out]
            n74 = call "Turn.vi"("mode"=w115, "Effort"=w117) -> ()  [unwired: 10 in]
          }
          frame #1 {
            n75 = call "Turn.vi"("mode"=1, "Effort"=0.0) -> ()  [unwired: 10 in]
          }
        }
      }
      frame "Intake" {
        n76 = flat-sequence {
          tunnel: w121 -> [w123]
          tunnel: w120 -> [w122]
          frame #0 {
            n77 = Wait (ms)(milliseconds to wait=w122) -> ()  [unwired: 1 out]
            n78 = call "Intake.vi"("Effort"=w123) -> ()  [unwired: 11 in]
          }
          frame #1 {
            n79 = call "Intake.vi"("Effort"=0.0) -> ()  [unwired: 11 in]
          }
        }
      }
      frame "Test" {
      }
      frame "Gear0" {
        n80 = flat-sequence {
          tunnel: w125 -> [w129]
          frame #0 {
            n81 = To Unsigned Byte Integer(number=w129) -> (unsigned 8bit integer=w128:u8)
            n82 = Number To Boolean Array(number=w128) -> (Boolean array=w127:bool[])
            n83 = Index Array(array=w127) -> (element=w126:bool)  [unwired: 1 in]
            n84 = call "Gear.vi"("Gear0?"=w126) -> ()  [unwired: 11 in]
          }
        }
      }
      frame "Gear1" {
        n85 = flat-sequence {
          tunnel: w130 -> [w134]
          frame #0 {
            n86 = To Unsigned Byte Integer(number=w134) -> (unsigned 8bit integer=w133:u8)
            n87 = Number To Boolean Array(number=w133) -> (Boolean array=w132:bool[])
            n88 = Index Array(array=w132) -> (element=w131:bool)  [unwired: 1 in]
            n89 = call "Gear.vi"("Gear1?"=w131) -> ()  [unwired: 11 in]
          }
        }
      }
      frame "Index" {
        n90 = flat-sequence {
          tunnel: w136 -> [w137]
          tunnel: w135 -> [_]
          frame #0 {
            n91 = Wait (ms)(milliseconds to wait=w137) -> ()  [unwired: 1 out]
            n92 = call "Index.vi"("Shoot"=TRUE ("Override?"), "Output"=-1.0) -> ()  [unwired: 10 in]
          }
          frame #1 {
            n93 = call "Index.vi"("Shoot"=FALSE ("Override?"), "Output"=0.0) -> ()  [unwired: 10 in]
          }
        }
      }
      frame "Climb" {
        n94 = flat-sequence {
          tunnel: w143 -> [w145]
          tunnel: w142 -> [w144]
          frame #0 {
            n95 = call "Climb.vi"("Effort"=w145) -> ()  [unwired: 11 in]
            n96 = Wait (ms)(milliseconds to wait=w144) -> ()  [unwired: 1 out]
          }
          frame #1 {
            n97 = call "Climb.vi"("Effort"=0.0) -> ()  [unwired: 11 in]
          }
        }
      }
      frame "Drive Encoder Reset" {
        n98 = while {
          stop <- w147 stop-if-true
          n99 = call <vilib>:"WPI_MotorControlRefNum Registry Get.vi"("refnum name"="Drive L1") -> ("error out"=w157:errorcluster, "MotorControlDevRef"=w152:T5)  [unwired: 9 in]
          n100 = call <vilib>:"WPI_MotorControlRefNum Registry Get.vi"("refnum name"="Drive R1") -> ("error out"=w162:errorcluster, "MotorControlDevRef"=w161:T5)  [unwired: 9 in]
          n101 = call <vilib>:"WPI_MotorControlRefNum Registry Get.vi"("refnum name"="Drive L1") -> ("error out"=w164:errorcluster, "MotorControlDevRef"=w165:T5)  [unwired: 9 in]
          n102 = call <vilib>:"WPI_MotorControlRefNum Registry Get.vi"("refnum name"="Drive R1") -> ("error out"=w154:errorcluster, "MotorControlDevRef"=w153:T5)  [unwired: 9 in]
          n103 = call <vilib>:"WPI_CANTalonSRX_SetSensorPosition.vi"("error in (no error)"=w162, "New Sensor Position"=0.0, "CAN Talon SRX Ref"=w161) -> ()  [unwired: 7 in, 2 out]
          n104 = call <vilib>:"WPI_CANTalonSRX_SetSensorPosition.vi"("error in (no error)"=w164, "New Sensor Position"=0.0, "CAN Talon SRX Ref"=w165) -> ()  [unwired: 7 in, 2 out]
          n105 = call <vilib>:"WPI_CANTalonSRX_GetStatus.vi"("error in (no error)"=w157, "CAN Talon SRX Ref"=w152) -> ("Talon SRX Status"=w155:T9)  [unwired: 7 in, 2 out]
          n106 = Unbundle By Name(w155) -> ("Encoder Position"=w150:dbl)
          n107 = call <vilib>:"WPI_CANTalonSRX_GetStatus.vi"("error in (no error)"=w154, "CAN Talon SRX Ref"=w153) -> ("Talon SRX Status"=w156:T9)  [unwired: 7 in, 2 out]
          n108 = Unbundle By Name(w156) -> ("Encoder Position"=w151:dbl)
          n109 = Equal To 0?(x=w150) -> (x = 0?=w149:bool)
          n110 = Equal To 0?(x=w151) -> (x = 0?=w148:bool)
          n111 = And(x=w149, y=w148) -> (x .and. y?=w147:bool)
        }
      }
      frame "Gyro Reset" {
        n112 = while {
          stop <- w168 stop-if-true
          w171 = 0.3
          n113 = call <vilib>:"WPI_GyroRefNum Registry Get.vi"("refnum name"="Gyro") -> ("error out"=w173:errorcluster, "GyroDevRef"=w174:T10)  [unwired: 9 in]
          n114 = global read "Global 2.vi" "Gyro"() -> (w169:dbl)
          n115 = call <vilib>:"WPI_GyroReset.vi"("error in"=w173, "GyroDevRef"=w174) -> ()  [unwired: 8 in, 2 out]
          n116 = Negate(x=w171) -> (-x=w170:dbl)
          n117 = In Range and Coerce(upper limit=w171, x=w169, lower limit=w170) -> (In Range?=w168:bool)  [unwired: 1 out]
        }
      }
    }
  }
